vi "Get Data Variant.vi"(8 "error in (no error)":errorcluster, 11 "UDP Tx Transfer Configuration in":refnum<class "UDP Transfer Tx Configuration.lvclass">=refnum) -> (0 "error out":errorcluster, 1 "data version":T1, 2 "data":variant, 3 "UDP Tx Transfer Configuration out":refnum<class "UDP Transfer Tx Configuration.lvclass">)   [LabVIEW 2020, in "UDP.lvlib" / "UDP Transfer Tx Configuration.lvclass"]
uses:
  UDP Transfer Tx Configuration.lvclass
  DSF Core.lvlibp/Typedefs/DSF Version Info.ctl
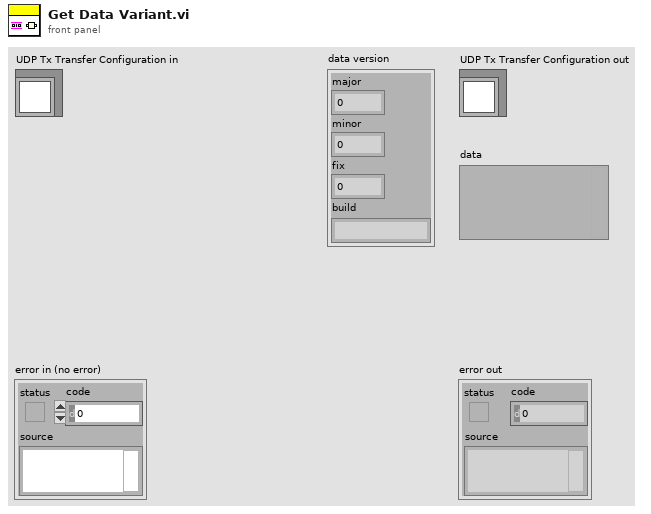
[diagram p1: front panel]
types:
  T1 = typedef "DSF Core.lvlibp/DSF Version Info.ctl" = cluster{"major":u32, "minor":u32, "fix":u32, "build":string}
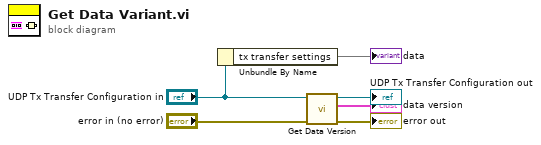
[diagram p0: block diagram]
diagram:
  n1 = Unbundle By Name("UDP Tx Transfer Configuration in") -> ("tx transfer settings"=→"data")
  n2 = call-dynamic "Get Data Version.vi"("error in (no error)"="error in (no error)", "UDP Tx Transfer Configuration in"="UDP Tx Transfer Configuration in") -> ("error out"=→"error out":errorcluster, "data version"=→"data version":T1, "UDP Tx Transfer Configuration out"=→"UDP Tx Transfer Configuration out":refnum<class "UDP Transfer Tx Configuration.lvclass">)  [unwired: 7 in]
